vi "Get Event-Reference Type Information.vi"() -> ()   [LabVIEW 2018, in "Scripting.lvlib"]
uses:
  Scripting.lvlib
  Event-Type-Information.ctl
  Error-Codes.ctl
  <vilib>/Utility/error.llb/Error Cluster From Error Code.vi
panel:
  out "error out":errorcluster
  out "Array":T1[](array[typedef])
  in  "error in (no error)":errorcluster
  in  "Events-Reference-Control-Path":path
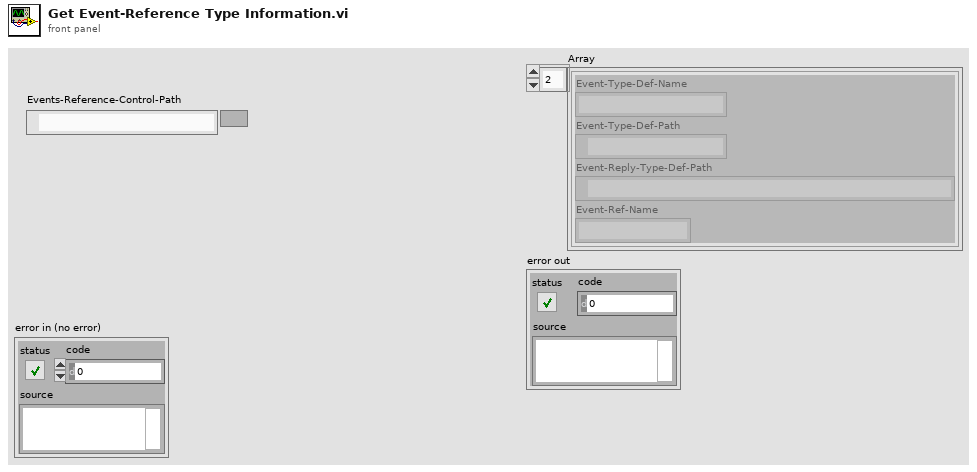
[diagram p1: front panel]
types:
  T1 = typedef "Scripting.lvlib/Event-Type-Information.ctl" = cluster{"Event-Type-Def-Name":string, "Event-Type-Def-Path":path, "Event-Reply-Type-Def-Path":path, "Event-Ref-Name":string}
  T2 = typedef "Scripting.lvlib/Error-Codes.ctl" = enum16{"EVENT_REF_TYPE_DEF_IS_NESTED", "EVENT_REF_TYPE_DEF_IS_EMPTY", "EVENT_REF_TYPE_DEF_INCLUDES_NON_REFS", "EVENT_REF_TYPE_INVALID_REPLY_REF", "EVENT_REF_TYPE_REPLY_IS_NOT_TYPE_DEF", "EVENT_REF_TYPE_DEF_IS_NOT_CLUSTER", "EVENT_REF_TYPE_DEF_INVALID_REQ_REPLY_TYPE"}
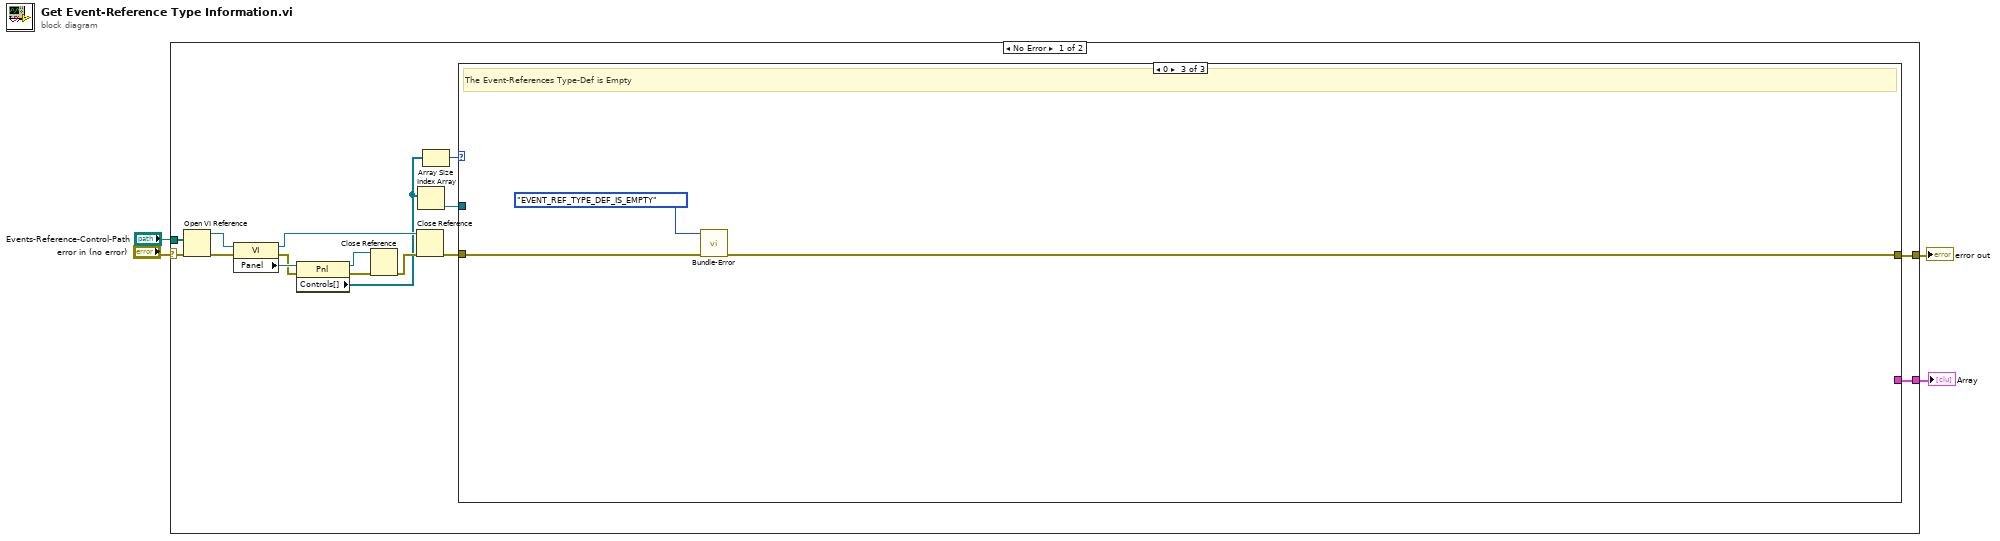
[diagram p0: block diagram]
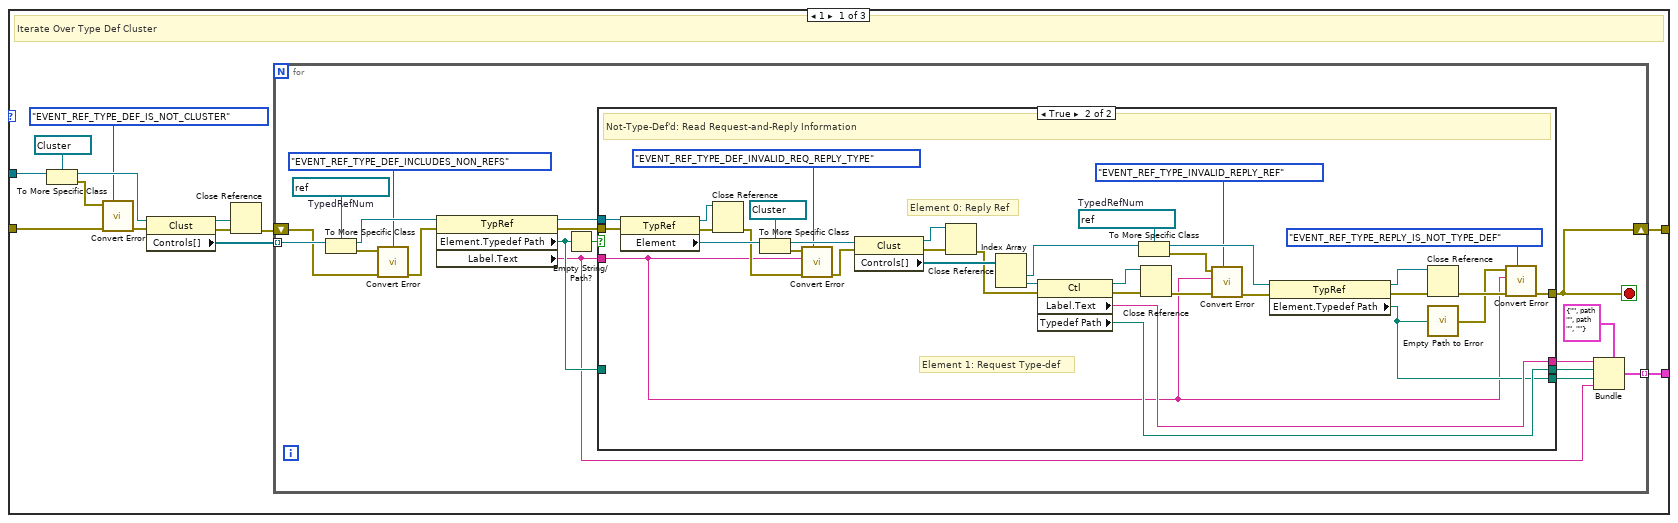
[diagram p2: hidden frame]
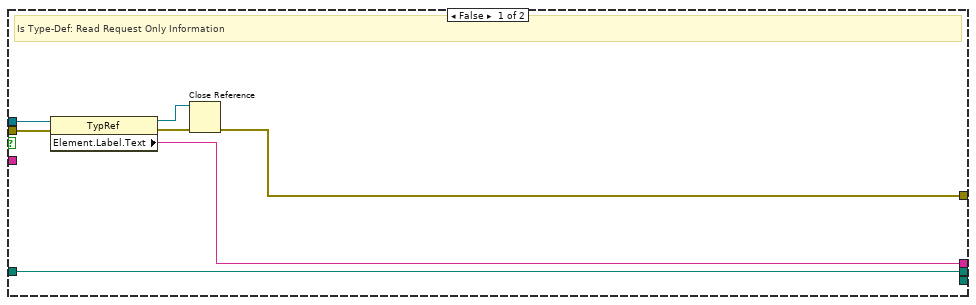
[diagram p3: hidden frame]
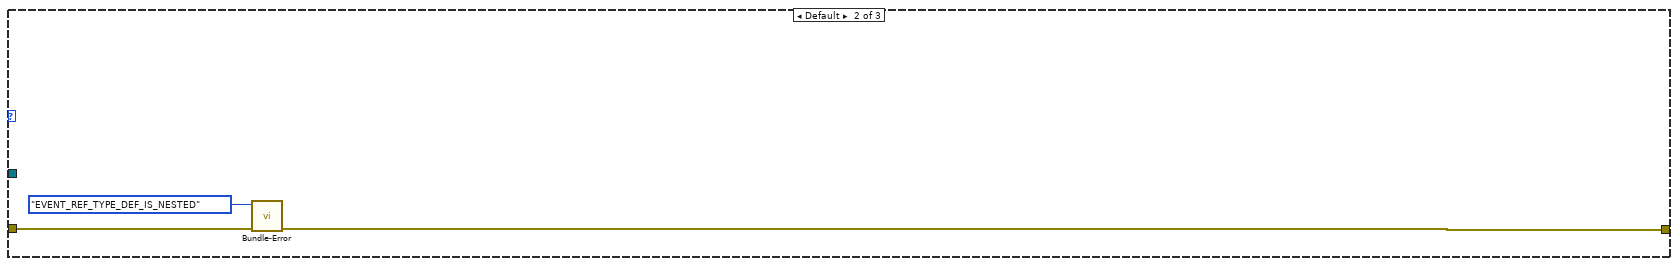
[diagram p4: hidden frame]
diagram:
  n1 = case shown="No Error" "error in (no error)" {
    selector: "error in (no error)" -> [w19 w100]
    tunnel: "Events-Reference-Control-Path" -> [w20 _]
    tunnel: [w8 _] -> w2
    tunnel: [w5 w100] -> w1
    frame No Error {
      n2 = Open VI Reference(vi path=w20, error in (no error)=w19) -> (vi reference=w16:refnum<vi>, error out=w17:errorcluster)  [unwired: 4 in]
      n3 = property class="VI"(reference=w16, error in=w17) -> (reference out=w14:refnum<vi>, error out=w9:errorcluster, "Panel"=w15:refnum<vi>)
      n4 = property class="Pnl"(reference=w15, error in=w9) -> (reference out=w13:refnum<vi>, error out=w12:errorcluster, "Controls[]"=w10:refnum<vi>[])
      n5 = Close Reference(reference=w13, error in (no error)=w12) -> (error out=w11:errorcluster)
      n6 = Close Reference(reference=w14, error in (no error)=w11) -> (error out=w6:errorcluster)
      n7 = Index Array(array=w10) -> (element=w7:refnum<vi>)  [unwired: 1 in]
      n8 = Array Size(array=w10) -> (size(s)=w18:i32)
      n9 = case shown="0" w18 {
        tunnel: [w32 w96 w98] -> w5
        tunnel: w7 -> [w29 _ _]
        tunnel: [w31 _ _] -> w8
        tunnel: w6 -> [w26 w94 w97]
        frame 1 {
          # "Iterate Over Type Def Cluster"
          n10 = To More Specific Class(target class=refnum<vi> refnum ("Type"), reference=w29) -> (specific class reference=w28:refnum<vi>, error out=w25:errorcluster)  [unwired: 1 in]
          n11 = call "Convert Error.vi"("Errors"=Error-Codes."EVENT_REF_TYPE_DEF_IS_NOT_CLUSTER", "error in (no error)"=w26, "Error Occured?"=w25) -> ("error out"=w27:errorcluster)  [unwired: 8 in]
          n12 = property class="Clust"(reference=w28, error in=w27) -> (reference out=w21:refnum<vi>, error out=w22:errorcluster, "Controls[]"=w33:refnum<vi>[])
          n13 = Close Reference(reference=w21, error in (no error)=w22) -> (error out=w23:errorcluster)
          n14 = for {
            tunnel: w33 -> [w51] mode=indexing
            shift-right: [w49] -> w32
            shift-left: w23 -> [w37]
            tunnel: [w48] -> w31 mode=indexing
            stop <- w49 stop-if-true
            w35 = refnum<vi> refnum  # TypedRefNum
            n15 = To More Specific Class(target class=w35, reference=w51) -> (specific class reference=w50:refnum<vi>, error out=w38:errorcluster)  [unwired: 1 in]
            n16 = call "Convert Error.vi"("Errors"=Error-Codes."EVENT_REF_TYPE_DEF_INCLUDES_NON_REFS", "error in (no error)"=w37, "Error Occured?"=w38) -> ("error out"=w36:errorcluster)  [unwired: 8 in]
            n17 = property class="TypRef"(reference=w50, error in=w36) -> (reference out=w46:refnum<vi>, error out=w45:errorcluster, "Element.Typedef Path"=w44:path, "Label.Text"=w40:string)
            n18 = Empty String/Path?(string/path=w44) -> (empty?=w47:bool)
            n19 = case shown="True" w47 {
              tunnel: w46 -> [w57 w93]
              tunnel: w45 -> [w58 w92]
              tunnel: w40 -> [_ w60]
              tunnel: [w52 w59] -> w49
              tunnel: [w55 w86] -> w42
              tunnel: [w56 w85] -> w43
              tunnel: [_ w84] -> w41
              tunnel: w44 -> [w55 _]
              frame False {
                # "Is Type-Def: Read Request Only Information"
                n20 = property class="TypRef"(reference=w57, error in=w58) -> (reference out=w54:refnum<vi>, error out=w53:errorcluster, "Element.Label.Text"=w56:string)
                n21 = Close Reference(reference=w54, error in (no error)=w53) -> (error out=w52:errorcluster)
              }
              frame True {
                w76 = refnum<vi> refnum  # TypedRefNum
                # "Element 1: Request Type-def"
                # "Element 0: Reply Ref"
                # "Not-Type-Def'd: Read Request-and-Reply Information"
                n22 = property class="TypRef"(reference=w93, error in=w92) -> (reference out=w83:refnum<vi>, error out=w90:errorcluster, "Element"=w91:refnum<vi>)
                n23 = Close Reference(reference=w83, error in (no error)=w90) -> (error out=w67:errorcluster)
                n24 = To More Specific Class(target class=refnum<vi> refnum ("Type"), reference=w91) -> (specific class reference=w89:refnum<vi>, error out=w65:errorcluster)  [unwired: 1 in]
                n25 = call "Convert Error.vi"("Errors"=Error-Codes."EVENT_REF_TYPE_DEF_INVALID_REQ_REPLY_TYPE", "error in (no error)"=w67, "error message (\"\")"=w60, "Error Occured?"=w65) -> ("error out"=w66:errorcluster)  [unwired: 7 in]
                n26 = property class="Clust"(reference=w89, error in=w66) -> (reference out=w79:refnum<vi>, error out=w80:errorcluster, "Controls[]"=w81:refnum<vi>[])
                n27 = Close Reference(reference=w79, error in (no error)=w80) -> (error out=w78:errorcluster)
                n28 = Index Array(array=w81) -> (element #1=w72:refnum<vi>, element #2=w77:refnum<vi>)  [unwired: 2 in]
                n29 = property class="Ctl"(reference=w77, error in=w78) -> (reference out=w87:refnum<vi>, error out=w88:errorcluster, "Label.Text"=w85:string, "Typedef Path"=w86:path)
                n30 = To More Specific Class(target class=w76, reference=w72) -> (specific class reference=w75:refnum<vi>, error out=w69:errorcluster)  [unwired: 1 in]
                n31 = Close Reference(reference=w87, error in (no error)=w88) -> (error out=w71:errorcluster)
                n32 = call "Convert Error.vi"("Errors"=Error-Codes."EVENT_REF_TYPE_INVALID_REPLY_REF", "error in (no error)"=w71, "error message (\"\")"=w60, "Error Occured?"=w69) -> ("error out"=w70:errorcluster)  [unwired: 7 in]
                n33 = property class="TypRef"(reference=w75, error in=w70) -> (reference out=w74:refnum<vi>, error out=w73:errorcluster, "Element.Typedef Path"=w84:path)
                n34 = Close Reference(reference=w74, error in (no error)=w73) -> (error out=w63:errorcluster)
                n35 = call "Empty Path to Error.vi"("Element.Typedef Path"=w84) -> ("error out"=w62:errorcluster)
                n36 = call "Convert Error.vi"("Errors"=Error-Codes."EVENT_REF_TYPE_REPLY_IS_NOT_TYPE_DEF", "error in (no error)"=w63, "error message (\"\")"=w60, "Error Occured?"=w62) -> ("error out"=w59:errorcluster)  [unwired: 7 in]
              }
            }
            n37 = Bundle(cluster=T1 {"Event-Type-Def-Name"="", "Event-Type-Def-Path"=path "", "Event-Reply-Type-Def-Path"=path "", "Event-Ref-Name"=""} ("output cluster"), "Event-Type-Def-Name"=w43, "Event-Type-Def-Path"=w42, "Event-Reply-Type-Def-Path"=w41, "Event-Ref-Name"=w40) -> (w48:T1)
          }
        }
        frame Default {
          n38 = call "Bundle-Error.vi"("error in (no error)"=w94, "Errors"=Error-Codes."EVENT_REF_TYPE_DEF_IS_NESTED") -> ("error out"=w96:errorcluster)  [unwired: 9 in]
        }
        frame 0 {
          # "The Event-References Type-Def is Empty"
          n39 = call "Bundle-Error.vi"("error in (no error)"=w97, "Errors"=Error-Codes."EVENT_REF_TYPE_DEF_IS_EMPTY") -> ("error out"=w98:errorcluster)  [unwired: 9 in]
        }
      }
    }
    frame Error {
    }
  }
  "Array" <- w2
  "error out" <- w1
